vi "Release.vi"(8 "error in (no error)":errorcluster, 11 "Publish JSON in":refnum<class "Publish JSON.lvclass">) -> (0 "error out":errorcluster)   [LabVIEW 2020, in "wamplv.lvlib" / "Publish JSON.lvclass"]
uses:
  Publish JSON.lvclass
  Publish JSON.lvclass/Publish JSON.ctl
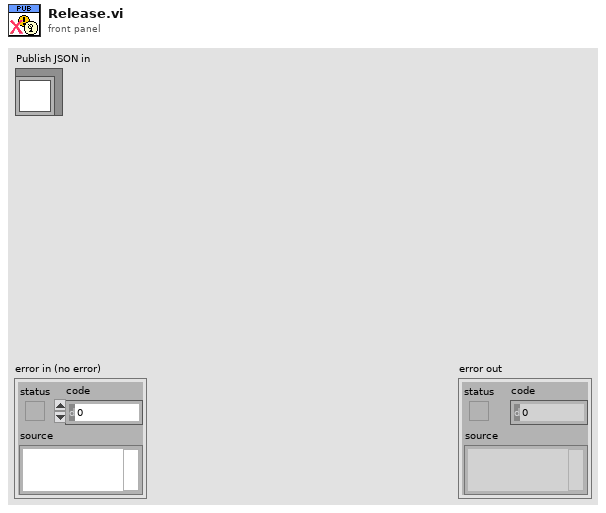
[diagram p1: front panel]
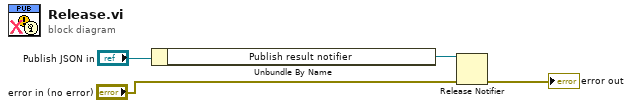
[diagram p0: block diagram]
diagram:
  n1 = Unbundle By Name("Publish JSON in") -> ("Publish result notifier"=w3:refnum<notifier>)
  n2 = Release Notifier(notifier=w3, error in (no error)="error in (no error)") -> (error out=→"error out":errorcluster)  [unwired: 1 in, 2 out]
